vi "GlobalVariables.vi"() -> ()   [LabVIEW 2019]
panel:
  out "Limelight Target Found?":dbl
  out "Previous Hood Setpoint Value":dbl
  out "Arm Height Pot Left":dbl
  out "Climber Control Value":dbl
  out "Positional Achieved?":bool
  out "Rotational Achieved?":bool
  out "Last Auto Gyro Value":dbl
  out "Shooter in range?":bool
  out "Hood Setpoint":dbl
  out "Hood Preset":enum16{"trench", "layup", "free track"}(ring)
  out "Hood Degrees":dbl
  out "RPM":dbl
  out "Arm Height Pot Right":dbl
  out "Turret Encoder Value":dbl
  out "Limelight LED State":dbl
  out "Turret Setpoint":dbl
  out "Turret Preset":enum16{"free track", "forward", "backward"}(ring)
  out "Shooter Wheels":enum16{"on", "off"}(ring)
  out "Arm Extension Encoder":dbl
  out "Arm Extension Setpoint":dbl
  out "Rotation Counter":dbl
  out "Control Panel Mode":enum16{"Rotational", "None", "Posistional"}(ring)
  out "Climber Mode":enum16{"Climb", "Control Panel"}(ring)
  out "Final Lock?":bool
  out "Intake State":enum16{"Idle", "Intake", "Spit"}(ring)
  out "Linear Acuator Setpoint":dbl
  out "Drive Gear":enum16{"high", "low"}(ring)
  out "Buddy Climb":enum16{"up", "deployed"}(ring)
  out "Climb Brake":enum16{"engaged", "off"}(ring)
  out "Arm Extension":T1(ring)
  out "Hopper Wheels":enum16{"on", "off"}(ring)
  out "Kicker Wheel":enum16{"on", "off", "reverse"}(ring)
  out "Arm Height":T2(ring)
  in  "Robot States":T3(ring)
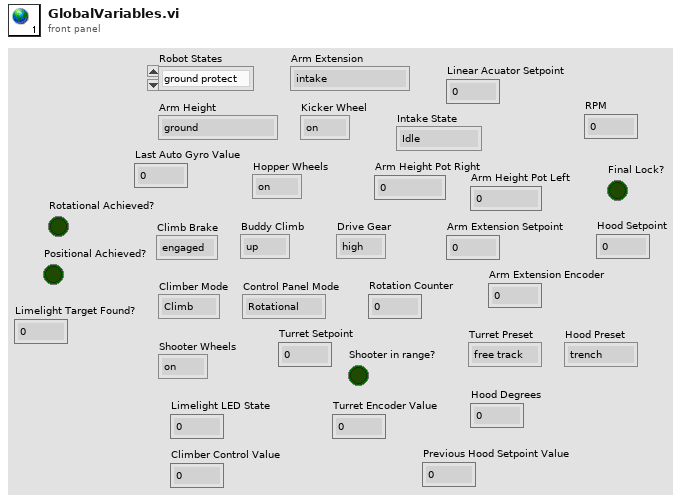
[diagram p1: front panel]
types:
  T1 = enum16{"intake", "protect", "control", "climb", "shooting"}
  T2 = enum16{"ground", "protect", "climb", "control panel"}
  T3 = enum16{"ground protect", "ground pickup", "control panel", "shooting", "climb", "unjam", "intake shoot"}
diagram:
